vi "Core Action.vi"(8 "error in (no error)":errorcluster, 10 "SECS-II Class":refnum<class "SECS-II Class.lvclass">, 11 "26-Host Requests to Enter OFF-Line in":refnum<class "26-Host Requests to Enter OFF-Line.lvclass">) -> (0 "error out":errorcluster, 2 "SECS-II Class Out":refnum<class "SECS-II Class.lvclass">, 3 "26-Host Requests to Enter OFF-Line out":refnum<class "26-Host Requests to Enter OFF-Line.lvclass">)   [LabVIEW 2020, in "SECS Scenarios.lvlib" / "26-Host Requests to Enter OFF-Line.lvclass"]
uses:
  26-Host Requests to Enter OFF-Line.lvclass
  D:/Dropbox/SECS/SECS_GEM v1.1.0/Com/SECS Scenarios/Scenarios Class/Scenarios Class.lvclass
  SECS Communication/SECS-II Class/SECS-II Class.lvclass
  SECS Communication/S1 Message Class/S1 Message Class.lvclass
  D:/Dropbox/SECS/SECS_GEM v1.1.0/Com/SECS Communication/SECS-II Class/SECS-II Class.lvclass
  Scenarios Class/Reply State.ctl
  Scenarios Class/Scenarios Class.lvclass/Scenarios Class.ctl
  Scenarios Class/Write Reply State.vi
  Scenarios Class/Read HSMS Class.vi
  SECS Communication/HSMS Class/HSMS Class.lvclass
  Scenarios Class/Scenarios Class.lvclass
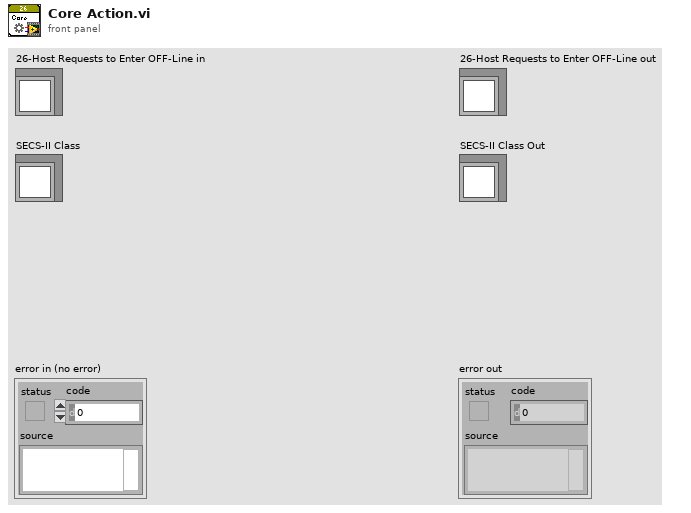
[diagram p1: front panel]
types:
  T1 = typedef "SECS Scenarios.lvlib/Scenarios Class.lvclass/Reply State.ctl" = enum16{"OK", "Illegal Data", "Unknown Stream", "Unknown Function", "Off-Line", "T3 Timeout", "Inner-Timeout"}
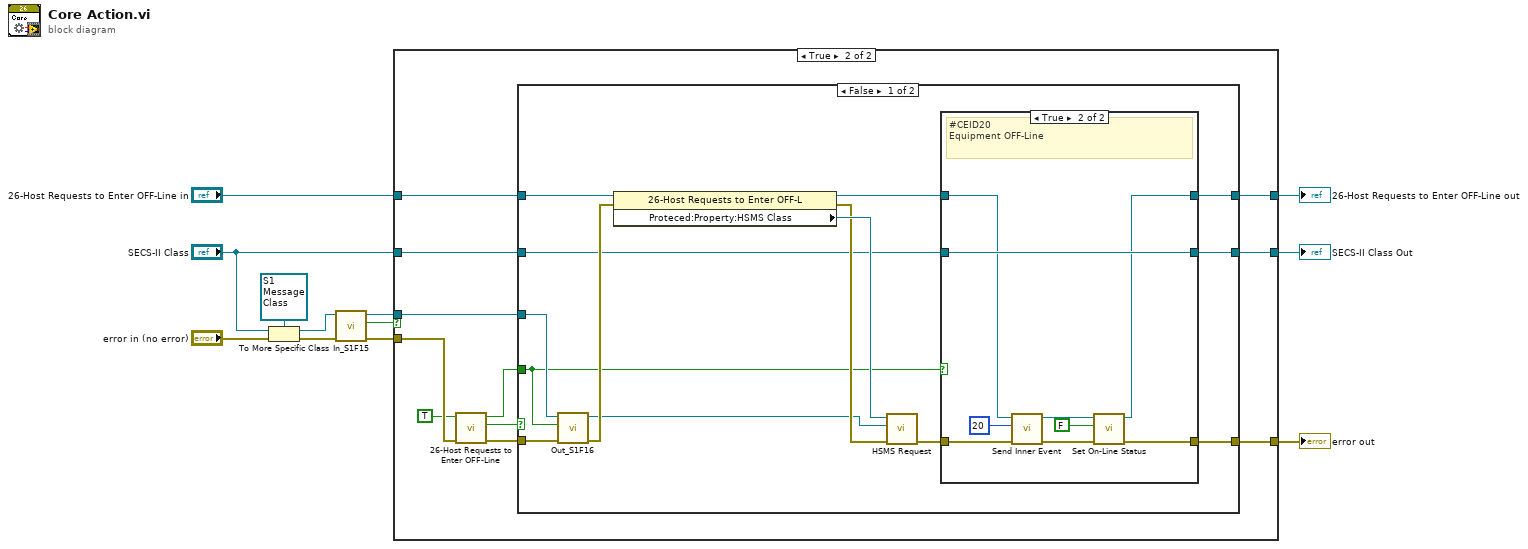
[diagram p0: block diagram]
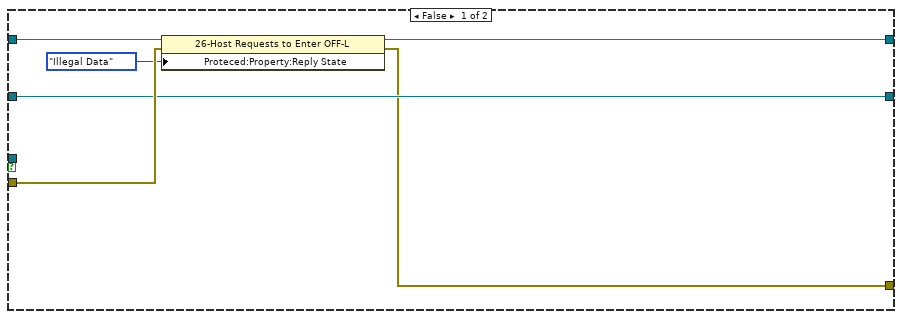
[diagram p2: hidden frame]
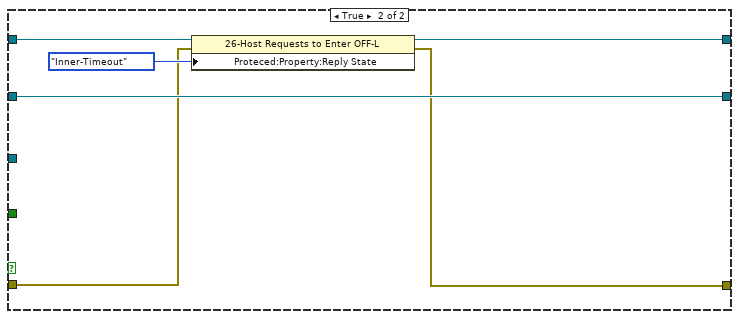
[diagram p4: hidden frame]
diagram:
  n1 = To More Specific Class(target class=refnum<class "S1 Message Class.lvclass"> refnum ("SECS Communication.lvlib:S1 Message Class.lvclass"), reference="SECS-II Class", error in="error in (no error)") -> (specific class reference=w11:refnum<class "S1 Message Class.lvclass">, error out=w12:errorcluster)
  n2 = call "In_S1F15.vi"("error in (no error)"=w12, "S1 Message Class in"=w11) -> ("error out"=w10:errorcluster, "OK?"=w1:bool, "S1 Message Class out"=w9:refnum<class "S1 Message Class.lvclass">)  [unwired: 7 in]
  n3 = case shown="True" w1 {
    tunnel: w10 -> [w17 w29]
    tunnel: w9 -> [_ w28]
    tunnel: "26-Host Requests to Enter OFF-Line in" -> [w18 w24]
    tunnel: [w13 w23] -> w5
    tunnel: [w15 w22] -> w4
    tunnel: "SECS-II Class" -> [w14 w21]
    tunnel: [w14 w20] -> w2
    frame False {
      n4 = property class="26-Host Requests to Enter OFF-L"(reference=w18, error in=w17, "Proteced:Property:Reply State"=Reply_State."Illegal Data" ("Reply State")) -> (reference out=w15:refnum<class "26-Host Requests to Enter OFF-Line.lvclass">, error out=w13:errorcluster)
    }
    frame True {
      n5 = call "26-Host Requests to Enter OFF-Line.vi"("error in (no error)"=w29, "Off-Line"=TRUE) -> ("error out"=w27:errorcluster, "Timeout?"=w26:bool, "Ack"=w25:bool)  [unwired: 7 in]
      n6 = case shown="False" w26 {
        tunnel: w24 -> [w43 w59]
        tunnel: w28 -> [w40 _]
        tunnel: [w34 w56] -> w23
        tunnel: [w32 w57] -> w22
        tunnel: w27 -> [w37 w58]
        tunnel: w25 -> [w35 _]
        tunnel: w21 -> [w31 w61]
        tunnel: [w30 w61] -> w20
        frame False {
          n7 = call "Out_S1F16.vi"("error in (no error)"=w37, "Ack"=w35, "S1 Message Class in"=w40) -> ("error out"=w39:errorcluster, "S1 Message Class out"=w38:refnum<class "S1 Message Class.lvclass">)  [unwired: 7 in]
          n8 = property class="26-Host Requests to Enter OFF-L"(reference=w43, error in=w39) -> (reference out=w33:refnum<class "26-Host Requests to Enter OFF-Line.lvclass">, error out=w41:errorcluster, "Proteced:Property:HSMS Class"=w42:refnum<class "HSMS Class.lvclass">)
          n9 = call "HSMS Request.vi"("error in (no error)"=w41, "SECS-II Class In"=w38, "HSMS Class in"=w42) -> ("error out"=w36:errorcluster)  [unwired: 7 in, 1 out]
          n10 = case shown="True" w35 {
            tunnel: w36 -> [w46 w51]
            tunnel: [w46 w52] -> w34
            tunnel: w33 -> [w45 w47]
            tunnel: [w45 w53] -> w32
            tunnel: w31 -> [w44 w55]
            tunnel: [w44 w55] -> w30
            frame False {
            }
            frame True {
              # "#CEID20\nEquipment OFF-Line"
              n11 = call "Send Inner Event.vi"("error in (no error)"=w51, "CEID"=u32 20, "Scenarios Class in"=w47) -> ("error out"=w49:errorcluster, "Scenarios Class out"=w48:refnum<class "26-Host Requests to Enter OFF-Line.lvclass">)  [unwired: 7 in]
              n12 = call "Set On-Line Status.vi"("error in (no error)"=w49, "On-Line"=FALSE ("On-Line Status"), "Scenarios Class in"=w48) -> ("error out"=w52:errorcluster, "Scenarios Class out"=w53:refnum<class "26-Host Requests to Enter OFF-Line.lvclass">)  [unwired: 7 in]
            }
          }
        }
        frame True {
          n13 = property class="26-Host Requests to Enter OFF-L"(reference=w59, error in=w58, "Proteced:Property:Reply State"=Reply_State."Inner-Timeout" ("Reply State")) -> (reference out=w57:refnum<class "26-Host Requests to Enter OFF-Line.lvclass">, error out=w56:errorcluster)
        }
      }
    }
  }
  "error out" <- w5
  "26-Host Requests to Enter OFF-Line out" <- w4
  "SECS-II Class Out" <- w2
